vi "OAT Shaft Centerline Plot Indicator.vi"() -> ()   [LabVIEW 2017]
doc: "Uses the Shaft Centerline plot to display the averaged positions of a shaft centeer on a customized picture control."
panel:
  out "Shaft Centerline Plot":picture
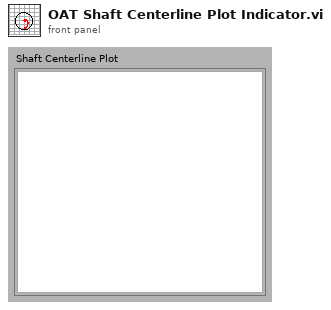
[diagram p1: front panel]
types:
  T1 = typedef "LVBoundsTypeDef.ctl" = cluster{"Width":u32, "Height":u32}
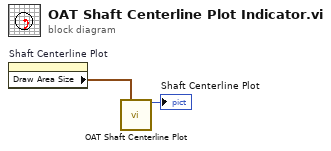
[diagram p0: block diagram]
diagram:
  n1 = property on="Shaft Centerline Plot" class="Pict"() -> ("Draw Area Size"=w2:T1)  [unwired: 2 in, 2 out]
  n2 = call <vilib>:"OAT Shaft Centerline Plot.vi"("picture\ndimensions (w,h)"=w2) -> ("new picture"=→"Shaft Centerline Plot":picture)  [unwired: 13 in, 1 out]
